vi "arm pid.vi"(1 "Setpoint":dbl, 2 "Autotune?":bool) -> (0 "Output":dbl)   [LabVIEW 2013]
uses:
  <vilib>/addons/control/pid/pid.llb/PID (DBL).vi
  <vilib>/addons/control/pid/NI_PID_autopid.lvlib
  <vilib>/addons/control/pid/NI_PID_pid.lvlib
panel:
  in  "autotuning parameters":T1={"controller type"=1, "relay cycles"=3, "relay amplitude"=1.0, "control specification"=2, "PV noise level"=0.1} {"controller type" items=["PID", "PI", "P"]; "control specification" items=["normal", "fast", "slow"]}
  in  "output range":cluster{"output high":dbl, "output low":dbl}={"output high"=1.0, "output low"=-1.0}
  in  "PID gains":T2={"proportional gain (Kc)"=1.0, "integral time (Ti, min)"=0.01, "derivative time (Td, min)"=0.0}
  # "Things needing Tuning"
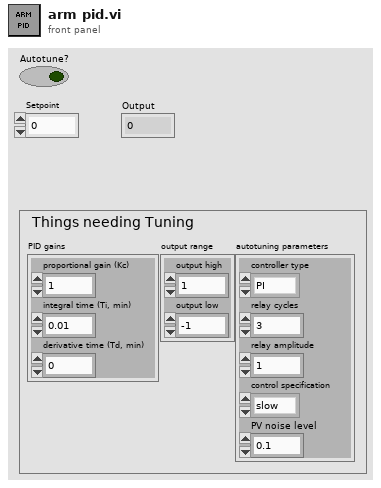
[diagram p1: front panel]
types:
  T1 = cluster{"controller type":u16, "relay cycles":i32, "relay amplitude":dbl, "control specification":u16, "PV noise level":dbl}
  T2 = cluster{"proportional gain (Kc)":dbl, "integral time (Ti, min)":dbl, "derivative time (Td, min)":dbl}
  T3 = typedef "WPI_EncoderDevRef.ctl" = cluster{"DevStatus":errorcluster, "EncoderIndex":T4, "CounterIndex":T5, "DistancePerCount":dbl, "Decoding Type":T6}
  T4 = typedef "FPGA_EncoderIdx.ctl" = enum8{"Enc 0", "Enc 1", "Enc 2", "Enc 3", "Invalid"}
  T5 = typedef "FPGA_CounterCtrSystemIndex.ctl" = enum8{"Ctr 0", "Ctr 1", "Ctr 2", "Ctr 3", "Ctr 4", "Ctr 5", "Ctr 6", "Ctr 7", "Invalid"}
  T6 = typedef "WPI_EncoderType.ctl" = enum16{"1x", "2x", "4x"}
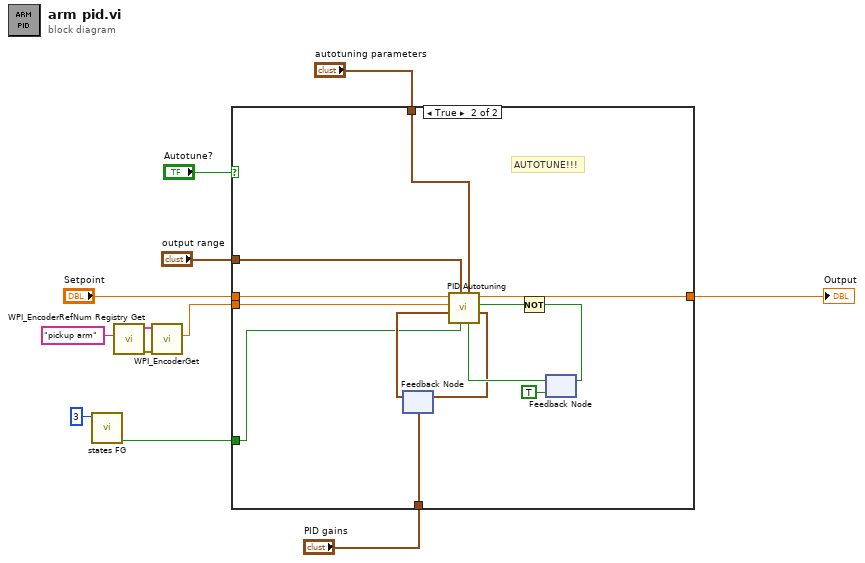
[diagram p0: block diagram]
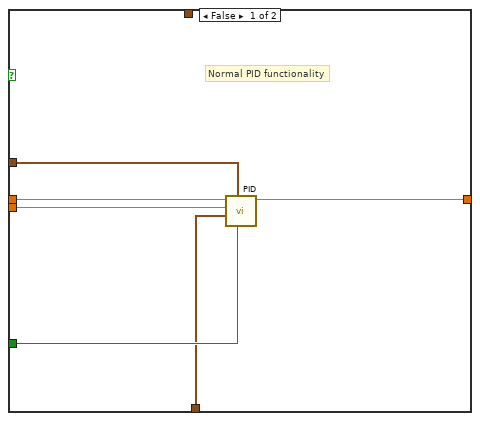
[diagram p2: hidden frame]
diagram:
  n1 = call "states FG.vi"("Loop ID"=3) -> ("first call?"=w4:bool)  [unwired: 7 in, 3 out]
  n2 = call <vilib>:"WPI_EncoderRefNum Registry Get.vi"("refnum name"="pickup arm") -> ("error out"=w10:errorcluster, "EncoderDevRef"=w9:T3)  [unwired: 9 in]
  n3 = call <vilib>:"WPI_EncoderGet.vi"("error in (no error)"=w10, "EncoderDevRef"=w9) -> ("Distance"=w8:dbl)  [unwired: 4 in, 5 out]
  n4 = case shown="True" "Autotune?" {
    tunnel: "Setpoint" -> [w18 w31]
    tunnel: [w17 w30] -> w11
    tunnel: w8 -> [w15 w23]
    tunnel: w4 -> [w16 w22]
    tunnel: "PID gains" -> [w14 w21]
    tunnel: "output range" -> [w13 w20]
    tunnel: "autotuning parameters" -> [_ w19]
    frame False {
      # "Normal PID functionality"
      n5 = call-poly <vilib>:"PID.vi"("reinitialize? (F)"=w16, "output range"=w13, "PID gains"=w14, "process variable"=w15, "setpoint"=w18) -> ("output"=w17:dbl)  [unwired: 5 in, 1 out]
    }
    frame True {
      # "AUTOTUNE!!!"
      n6 = feedback #1(w21) -> (w24:T2)
      n7 = feedback #2(TRUE) -> (w27:bool)
      n8 = call <vilib>:"PID Autotuning.vi"("autotune? (F)"=w27, "autotuning parameters"=w19, "reinitialize? (F)"=w22, "output range"=w20, "PID gains"=w24, "process variable"=w23, "setpoint"=w31) -> ("PID gains out"=w25:T2, "tuning completed?"=w29:bool, "output"=w30:dbl)  [unwired: 1 in, 1 out]
      n9 = feedback-in #1(w25) -> ()
      n10 = Not(x=w29) -> (.not. x?=w28:bool)
      n11 = feedback-in #2(w28) -> ()
    }
  }
  "Output" <- w11
